vi "FestoCPX.Station.ProdPresent.Group.vi"(8 "error in":errorcluster, 10 "Prod Present":T2) -> (0 "error out":errorcluster, 2 "Prod Present GUI":T1)   [LabVIEW 2016]
uses:
  FestoCPX.Station.ProdPresent.ctl
  FestoCPX.Station.ProdPresentGUI.ctl
  Station/Station.Global.vi
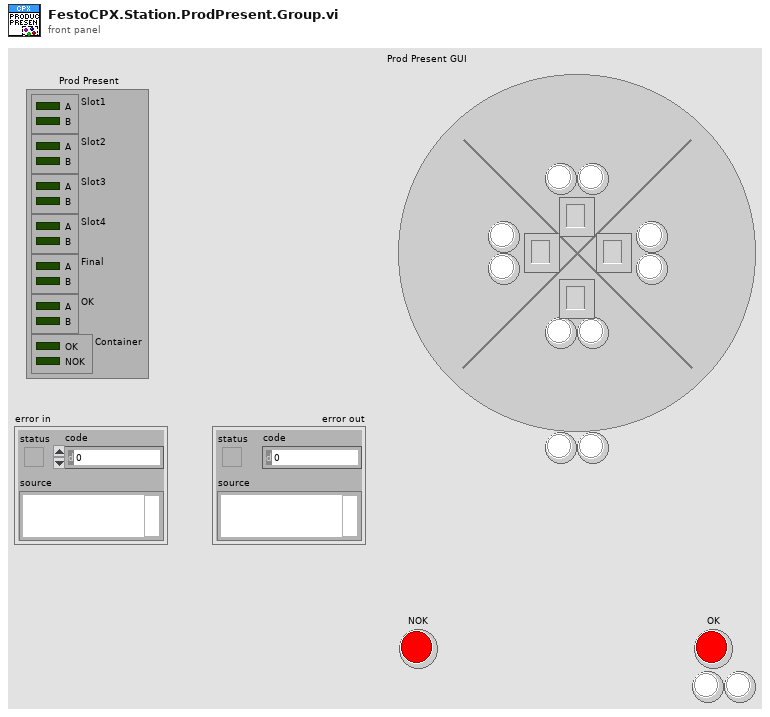
[diagram p1: front panel]
types:
  T1 = typedef "FestoCPX.Station.ProdPresentGUI.ctl" = cluster{"ProdPresentSlotRightA":bool, "ProdPresentSlotRightB":bool, "ProdPresentSlotTopA":bool, "ProdPresentSlotTopB":bool, "ProdPresentSlotLeftA":bool, "ProdPresentSlotLeftB":bool, "ProdPresentSlotBottomA":bool, "ProdPresentSlotBottomB":bool, "SlotNoRight":u8, "SlotNoTop":u8, "SlotNoLeft":u8, "SlotNoBottom":u8, "ProdFinalA":bool, "ProdFinalB":bool, "ProdFinalA 2":bool, "ProdFinalB 2":bool, "ProdContainerOK":bool, "ProdContainerNOK":bool}
  T2 = typedef "FestoCPX.Station.ProdPresent.ctl" = cluster{"Slot1":cluster{"A":bool, "B":bool}, "Slot2":cluster{"A":bool, "B":bool}, "Slot3":cluster{"A":bool, "B":bool}, "Slot4":cluster{"A":bool, "B":bool}, "Final":cluster{"A":bool, "B":bool}, "OK":cluster{"A":bool, "B":bool}, "Container":cluster{"OK":bool, "NOK":bool}}
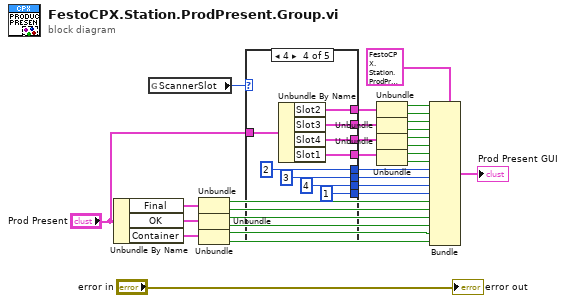
[diagram p0: block diagram]
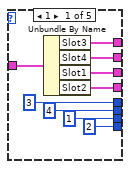
[diagram p2: hidden frame]
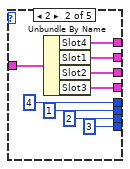
[diagram p3: hidden frame]
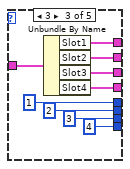
[diagram p4: hidden frame]
diagram:
  n1 = Unbundle By Name("Prod Present") -> ("Final"=w25:cluster{"A":bool, "B":bool}, "OK"=w11:cluster{"A":bool, "B":bool}, "Container"=w6:cluster{"OK":bool, "NOK":bool})
  n2 = global read "Station.Global.vi" "ScannerSlot"() -> (w2:i32)
  n3 = Unbundle(w25) -> ("A"=w29:bool, "B"=w28:bool)
  n4 = Unbundle(w11) -> ("A"=w27:bool, "B"=w26:bool)
  n5 = Unbundle(w6) -> ("OK"=w5:bool, "NOK"=w4:bool)
  n6 = case shown="4" w2 {
    tunnel: [u8 3 ("SlotNoLeft") u8 4 ("SlotNoLeft") u8 1 ("SlotNoLeft") u8 2 ("SlotNoLeft") _] -> w1
    tunnel: [u8 4 ("SlotNoLeft") u8 1 ("SlotNoLeft") u8 2 ("SlotNoLeft") u8 3 ("SlotNoLeft") _] -> w24
    tunnel: [u8 1 ("SlotNoLeft") u8 2 ("SlotNoLeft") u8 3 ("SlotNoLeft") u8 4 ("SlotNoLeft") _] -> w23
    tunnel: [u8 2 ("SlotNoLeft") u8 3 ("SlotNoLeft") u8 4 ("SlotNoLeft") u8 1 ("SlotNoLeft") _] -> w22
    tunnel: [w34 w43 w52 w62 _] -> w21
    tunnel: [w33 w42 w51 w61 _] -> w8
    tunnel: [w32 w41 w50 w60 _] -> w9
    tunnel: [w31 w40 w49 w59 _] -> w10
    tunnel: "Prod Present" -> [w35 w44 w53 w58 _]
    frame 1 {
      n7 = Unbundle By Name(w35) -> ("Slot3"=w34:cluster{"A":bool, "B":bool}, "Slot4"=w33:cluster{"A":bool, "B":bool}, "Slot1"=w32:cluster{"A":bool, "B":bool}, "Slot2"=w31:cluster{"A":bool, "B":bool})
    }
    frame 2 {
      n8 = Unbundle By Name(w44) -> ("Slot4"=w43:cluster{"A":bool, "B":bool}, "Slot1"=w42:cluster{"A":bool, "B":bool}, "Slot2"=w41:cluster{"A":bool, "B":bool}, "Slot3"=w40:cluster{"A":bool, "B":bool})
    }
    frame 3 {
      n9 = Unbundle By Name(w53) -> ("Slot1"=w52:cluster{"A":bool, "B":bool}, "Slot2"=w51:cluster{"A":bool, "B":bool}, "Slot3"=w50:cluster{"A":bool, "B":bool}, "Slot4"=w49:cluster{"A":bool, "B":bool})
    }
    frame 4 {
      n10 = Unbundle By Name(w58) -> ("Slot2"=w62:cluster{"A":bool, "B":bool}, "Slot3"=w61:cluster{"A":bool, "B":bool}, "Slot4"=w60:cluster{"A":bool, "B":bool}, "Slot1"=w59:cluster{"A":bool, "B":bool})
    }
    frame Default {
    }
  }
  n11 = Unbundle(w21) -> ("A"=w20:bool, "B"=w19:bool)
  n12 = Unbundle(w8) -> ("A"=w18:bool, "B"=w17:bool)
  n13 = Unbundle(w9) -> ("A"=w16:bool, "B"=w15:bool)
  n14 = Unbundle(w10) -> ("A"=w14:bool, "B"=w13:bool)
  n15 = Bundle(cluster=T1 {"ProdPresentSlotRightA"=FALSE, "ProdPresentSlotRightB"=FALSE, "ProdPresentSlotTopA"=FALSE, "ProdPresentSlotTopB"=FALSE, "ProdPresentSlotLeftA"=FALSE, "ProdPresentSlotLeftB"=FALSE, "ProdPresentSlotBottomA"=FALSE, "ProdPresentSlotBottomB"=FALSE, "SlotNoRight"=0, "SlotNoTop"=0, "SlotNoLeft"=0, "SlotNoBottom"=0, "ProdFinalA"=FALSE, "ProdFinalB"=FALSE, "ProdFinalA 2"=FALSE, "ProdFinalB 2"=FALSE, "ProdContainerOK"=FALSE, "ProdContainerNOK"=FALSE} ("Prod Present GUI"), "ProdPresentSlotRightA"=w20, "ProdPresentSlotRightB"=w19, "ProdPresentSlotTopA"=w18, "ProdPresentSlotTopB"=w17, "ProdPresentSlotLeftA"=w16, "ProdPresentSlotLeftB"=w15, "ProdPresentSlotBottomA"=w14, "ProdPresentSlotBottomB"=w13, "SlotNoRight"=w1, "SlotNoTop"=w24, "SlotNoLeft"=w23, "SlotNoBottom"=w22, "ProdFinalA"=w29, "ProdFinalB"=w28, "ProdFinalA 2"=w27, "ProdFinalB 2"=w26, "ProdContainerOK"=w5, "ProdContainerNOK"=w4) -> (→"Prod Present GUI":T1)
  "error out" <- "error in"
